vi "FTW-Actor-Log-Event.vi"(0 "FTW Actor Instance":refnum<class "FTW-ActorInstance.lvclass">, 5 "Event Type":string, 7 "Event Data":string, 9 "Source (unwired for call chain)":string="CallChain", 11 "error in":errorcluster) -> (4 "FTW Actor Instance out":refnum<class "FTW-ActorInstance.lvclass">, 6 "Serialized Event":string, 15 "error out":errorcluster)   [LabVIEW 2012, in "FTW-Actor.lvlib" / "FTW-ActorInstance.lvclass"]
uses:
  FTW-ActorInstance.lvclass
  FTW-ActorInstance.lvclass/FTW-ActorInstance.ctl
  EventLogger/FTW-Logger.lvclass
panel:
  # "Inputs"
  # "Outputs"
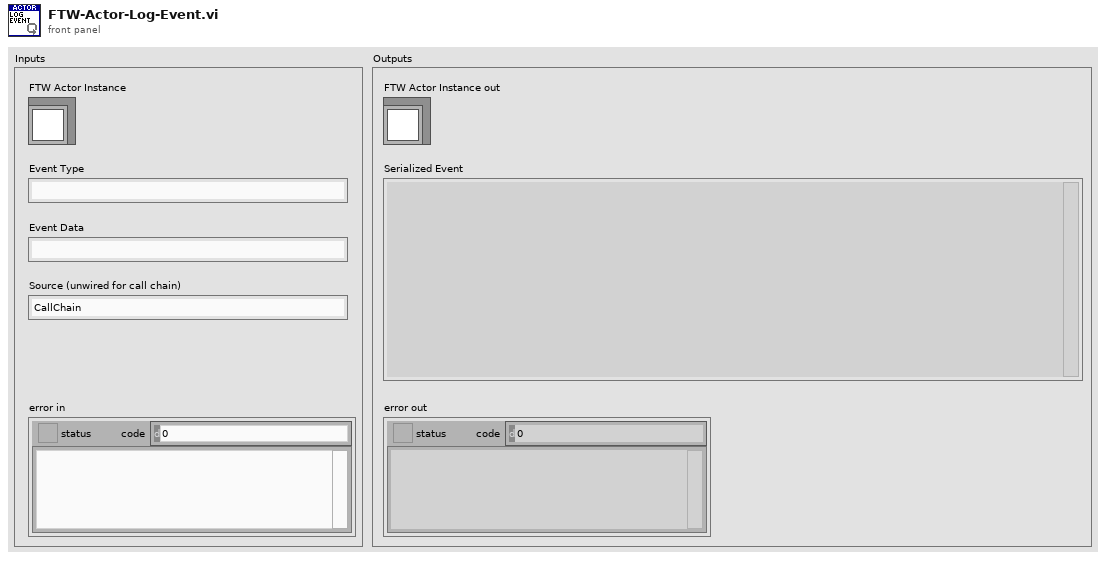
[diagram p1: front panel]
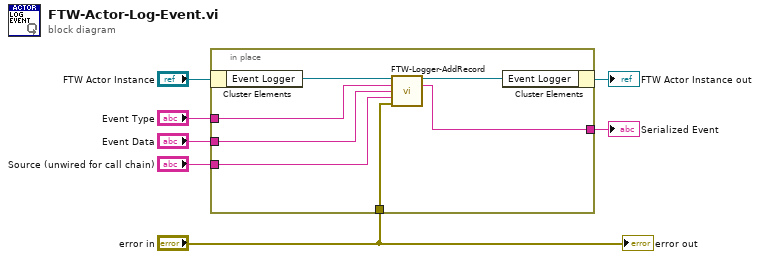
[diagram p0: block diagram]
diagram:
  n1 = in-place {
    in-place-border: "error in" -> [w14]
    in-place-border: [w11] -> w5
    in-place-border: "Event Type" -> [w10]
    in-place-border: "Event Data" -> [w9]
    in-place-border: "Source (unwired for call chain)" -> [w8]
    n2 = in-place-cluster #1("FTW Actor Instance") -> ("Event Logger"=w13:refnum<class "FTW-Logger.lvclass">)
    n3 = call "FTW-Logger-AddRecord.vi"("FTW Logger Connector"=w13, "Event Type"=w10, "Event Data"=w9, "Source (unwired for call chain)"=w8, "error in"=w14) -> ("FTW Logger Connector out"=w12:refnum<class "FTW-Logger.lvclass">, "Serialized Event"=w11:string)  [unwired: 8 in, 1 out]
    n4 = in-place-cluster #1("Event Logger"=w12) -> (→"FTW Actor Instance out":refnum<class "FTW-ActorInstance.lvclass">)
  }
  "Serialized Event" <- w5
  "error out" <- "error in"
